vi "Open Configuration File.vi"(7 "Fileopts":T1={"Name/Value delimiter (\"=\")"="=", "Comment delimiter (\";\")"=";"}, 8 "error in (no error)":errorcluster, 10 "create file if necessary (T)":bool=TRUE, 11 "configuration file path":path) -> (0 "error out":errorcluster, 2 "file created?":bool, 3 "Configuration Reference":refnum<data-value>)   [LabVIEW 2012, in "configlib.lvlib"]
uses:
  configlib.lvlib
  Configuration File Definition.ctl
  File Options.ctl
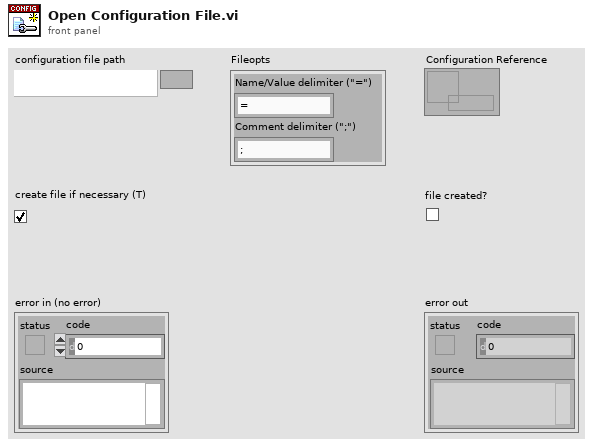
[diagram p1: front panel]
types:
  T1 = typedef "configlib.lvlib/File Options.ctl" = cluster{"Name/Value delimiter (\"=\")":string, "Comment delimiter (\";\")":string}
  T2 = typedef "configlib.lvlib/Configuration File Definition.ctl" = cluster{"dirty":bool, "path":path, "Fileopts":T1, "Section Lookup":variant, "Key Lookup":variant, "Raw File":string[]}
  T3 = enum16{"open", "replace", "create", "open or create", "replace or create", "replace or create with confirmation"}
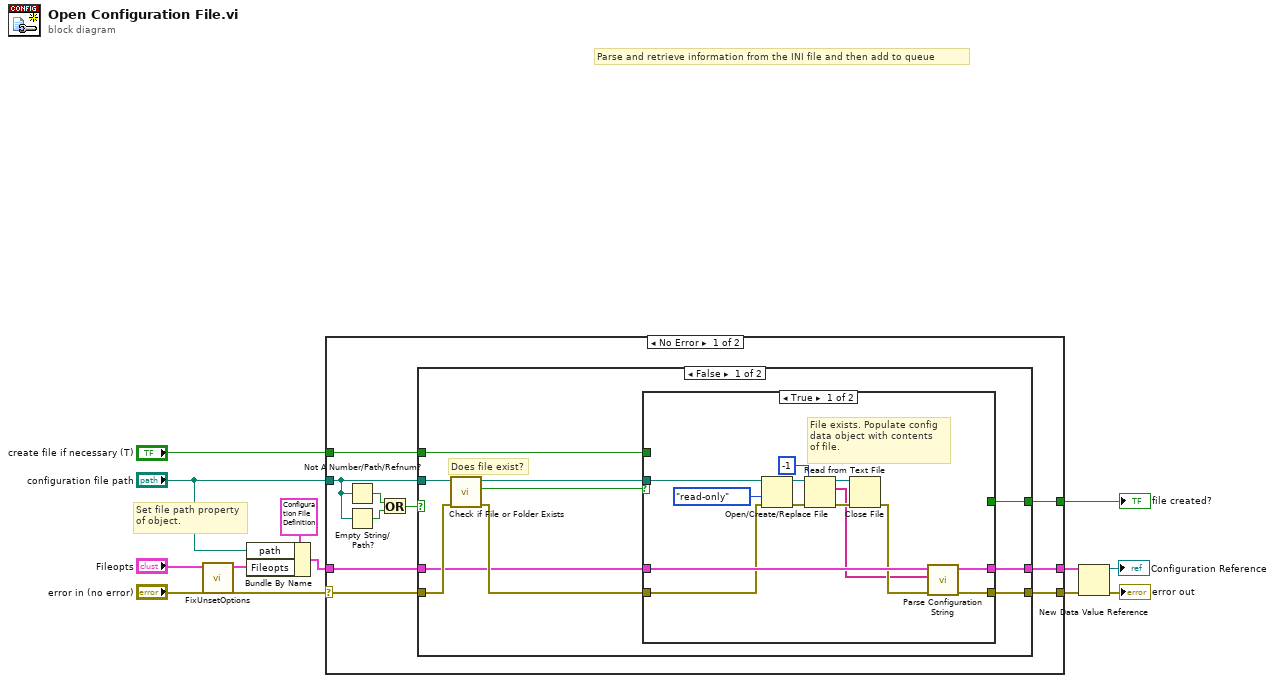
[diagram p0: block diagram]
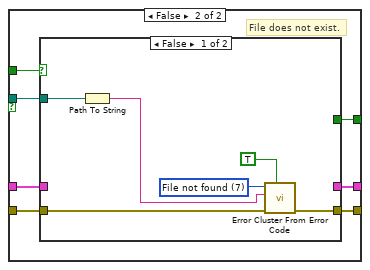
[diagram p2: hidden frame]
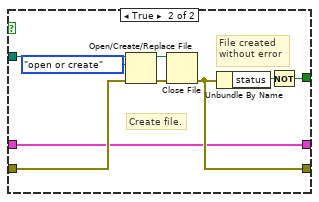
[diagram p3: hidden frame]
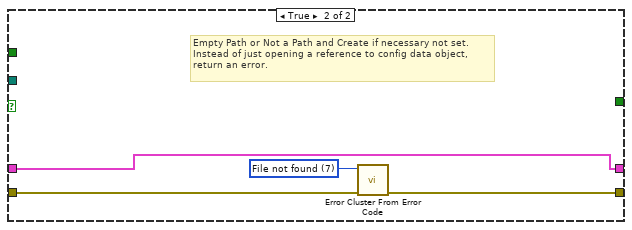
[diagram p4: hidden frame]
diagram:
  # "Parse and retrieve information from the INI file and then add to queue"
  # "Set file path property\nof object."
  n1 = call "FixUnsetOptions.vi"("Fileopts in"="Fileopts") -> ("Fileopts out"=w1:T1)  [unwired: 10 in]
  n2 = Bundle By Name(cluster=T2 {"dirty"=FALSE, "path"=path "", "Fileopts"={"Name/Value delimiter (\"=\")"="", "Comment delimiter (\";\")"=""}, "Section Lookup"=variant, "Key Lookup"=variant, "Raw File"=[]}, "path"="configuration file path", "Fileopts"=w1) -> (w8:T2)
  n3 = case shown="No Error" "error in (no error)" {
    selector: "error in (no error)" -> [w18 w73]
    tunnel: [w16 w73] -> w7
    tunnel: "configuration file path" -> [w17 _]
    tunnel: "create file if necessary (T)" -> [w19 _]
    tunnel: [w15 _] -> w10
    tunnel: w8 -> [w14 w72]
    tunnel: [w13 w72] -> w5
    frame No Error {
      n4 = Not A Number/Path/Refnum?(number/path/refnum=w17) -> (NaN/Path/Refnum?=w21:bool)
      n5 = Empty String/Path?(string/path=w17) -> (empty?=w22:bool)
      n6 = Or(x=w21, y=w22) -> (x .or. y?=w20:bool)
      n7 = case shown="False" w20 {
        tunnel: [w32 w71] -> w16
        tunnel: w17 -> [w28 _]
        tunnel: w19 -> [w31 _]
        tunnel: w18 -> [w27 w69]
        tunnel: [w30 _] -> w15
        tunnel: w14 -> [w24 w68]
        tunnel: [w23 w68] -> w13
        frame False {
          # "Does file exist?"
          n8 = call <vilib>:"Check if File or Folder Exists.vi"("error in (no error)"=w27, "path"=w28) -> ("error out"=w26:errorcluster, "file or folder exists?"=w29:bool, "dup path"=w25:path)  [unwired: 7 out]
          n9 = case shown="True" w29 {
            tunnel: [w40 w51] -> w32
            tunnel: w25 -> [w36 w52]
            tunnel: w31 -> [_ w50]
            tunnel: [_ w49] -> w30
            tunnel: w26 -> [w37 w48]
            tunnel: w24 -> [w42 w47]
            tunnel: [w41 w46] -> w23
            frame True {
              # "File exists. Populate config\ndata object with contents\nof file."
              n10 = Open/Create/Replace File(file path (use dialog)=w36, error in=w37, access (0:read/write)=enum16{"read/write", "read-only", "write-only"}."read-only") -> (refnum out=w43:refnum<file>, error out=w35:errorcluster)  [unwired: 4 out]
              n11 = Read from Text File(file (use dialog)=w43, count=-1, error in=w35) -> (refnum out=w45:refnum<file>, text=w33:string[], error out=w39:errorcluster)  [unwired: 2 out]
              n12 = Close File(refnum=w45, error in=w39) -> (error out=w38:errorcluster)  [unwired: 1 out]
              n13 = call "Parse Configuration String.vi"("error in (no error)"=w38, "Configuration String Lines"=w33, "Configuration In"=w42) -> ("error out"=w40:errorcluster, "Configuration Out"=w41:T2)  [unwired: 7 in]
            }
            frame False {
              # "File does not exist."
              n14 = case shown="False" w50 {
                tunnel: w52 -> [w54 w67]
                tunnel: [w57 w61] -> w51
                tunnel: [_ w60] -> w49
                tunnel: w48 -> [w56 w63]
                tunnel: w47 -> [_ w59]
                tunnel: [_ w59] -> w46
                frame False {
                  w58 = u16 7 items=["No error", "Argument error", "Memory is full", "Out of zone", "End of file", "File already open", "Generic file I/O error", "File not found", "File permission error", "Disk is full", "Duplicate path", "Too many files open", "System feature not enabled", "Resource file not found", "Cannot add resource", "Resource not found", "Image not found", "Image memory error", "Pen does not exist", "Config type invalid", "Config token not found", "Config parse error", "Config memory error", "Bad external code format", "Bad external code offset", "External code not present", "Null window", "Destroy window error", "Null menu", "Print aborted", "Bad print record", "Print driver error", "Windows error during printing", "Memory error during printing", "Print dialog error", "Generic print error", "Invalid device refnum", "Device not found", "Device parameter error", "Device unit error", "Cannot open device", "Device call aborted", "Generic error", "Cancelled by user", "Object ID too low", "Object ID too high", "Object not in heap", "Unknown heap", "Unknown object (invalid DefProc)", "Unknown object (DefProc not in table)", "Message out of range", "Invalid (null) method", "Unknown message", "Manager call not supported", "Bad address", "Network operation in progress", "Network operation timed out", "Connection is busy", "Network attribute not supported", "Network error", "Address in use", "System out of memory", "Connection aborted", "Connection refused", "Not connected", "Already connected", "Connection closed", "Initialization error (interapplication manager)", "Bad occurrence", "Wait on unbound occurrence handler", "Occurrence queue overflow", "Datalog type conflict", "Unused", "Unrecognized type (interapplication manager)", "Memory corrupt", "Failed to make temporary DLL", "Old CIN version", "Drag socket not found", "Failed to load drop-object", "Failed to register OLE object", "Failed to release OLE object", "Format specifier type mismatch", "Unknown format specifier", "Too few format specifiers", "Too many format specifiers", "Scan failed", "Newer CIN version", "OLE Convert", "Runtime menu error", "Password tampered", "Unknown error code"]
                  n15 = Path To String(path=w54) -> (string=w53:string)
                  n16 = call <vilib>:"Error Cluster From Error Code.vi"("show call chain? (False)"=TRUE, "error in (no error)"=w56, "error message (\"\")"=w53, "error code (0)"=w58) -> ("error out"=w57:errorcluster)  [unwired: 5 out]
                }
                frame True {
                  # "File created\nwithout error"
                  # "Create file."
                  n17 = Open/Create/Replace File(file path (use dialog)=w67, error in=w63, operation (0:open)=T3."open or create") -> (refnum out=w65:refnum<file>, error out=w66:errorcluster)  [unwired: 4 out]
                  n18 = Close File(refnum=w65, error in=w66) -> (error out=w61:errorcluster)  [unwired: 1 out]
                  n19 = Unbundle By Name(w61) -> ("status"=w62:bool)
                  n20 = Not(x=w62) -> (.not. x?=w60:bool)
                }
              }
            }
          }
        }
        frame True {
          w70 = u16 7 items=["No error", "Argument error", "Memory is full", "Out of zone", "End of file", "File already open", "Generic file I/O error", "File not found", "File permission error", "Disk is full", "Duplicate path", "Too many files open", "System feature not enabled", "Resource file not found", "Cannot add resource", "Resource not found", "Image not found", "Image memory error", "Pen does not exist", "Config type invalid", "Config token not found", "Config parse error", "Config memory error", "Bad external code format", "Bad external code offset", "External code not present", "Null window", "Destroy window error", "Null menu", "Print aborted", "Bad print record", "Print driver error", "Windows error during printing", "Memory error during printing", "Print dialog error", "Generic print error", "Invalid device refnum", "Device not found", "Device parameter error", "Device unit error", "Cannot open device", "Device call aborted", "Generic error", "Cancelled by user", "Object ID too low", "Object ID too high", "Object not in heap", "Unknown heap", "Unknown object (invalid DefProc)", "Unknown object (DefProc not in table)", "Message out of range", "Invalid (null) method", "Unknown message", "Manager call not supported", "Bad address", "Network operation in progress", "Network operation timed out", "Connection is busy", "Network attribute not supported", "Network error", "Address in use", "System out of memory", "Connection aborted", "Connection refused", "Not connected", "Already connected", "Connection closed", "Initialization error (interapplication manager)", "Bad occurrence", "Wait on unbound occurrence handler", "Occurrence queue overflow", "Datalog type conflict", "Unused", "Unrecognized type (interapplication manager)", "Memory corrupt", "Failed to make temporary DLL", "Old CIN version", "Drag socket not found", "Failed to load drop-object", "Failed to register OLE object", "Failed to release OLE object", "Format specifier type mismatch", "Unknown format specifier", "Too few format specifiers", "Too many format specifiers", "Scan failed", "Newer CIN version", "OLE Convert", "Runtime menu error", "Password tampered", "Unknown error code"]
          # "Empty Path or Not a Path and Create if necessary not set.\nInstead of just opening a reference to config data object,\nreturn an error."
          n21 = call <vilib>:"Error Cluster From Error Code.vi"("error in (no error)"=w69, "error code (0)"=w70) -> ("error out"=w71:errorcluster)  [unwired: 1 in, 6 out]
        }
      }
    }
    frame Error {
    }
  }
  "file created?" <- w10
  n22 = New Data Value Reference(data value=w5, error in=w7) -> (data value reference=→"Configuration Reference":refnum<data-value>, error out=→"error out":errorcluster)
